vi "Panel.vi"(1 "枚举":enum16{"loop", "back", "advance", "clear"}(ring), 2 "vi reference In":refnum<vi>) -> (0 "vi reference Out":refnum<vi>)   [LabVIEW 2015]
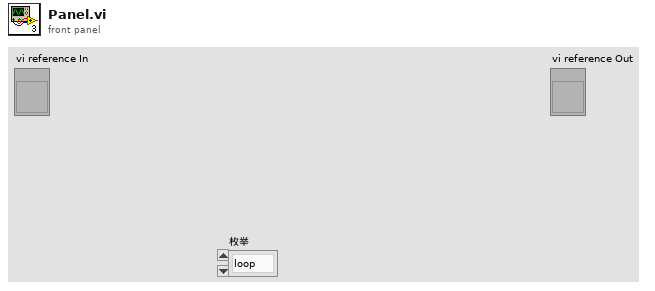
[diagram p1: front panel]
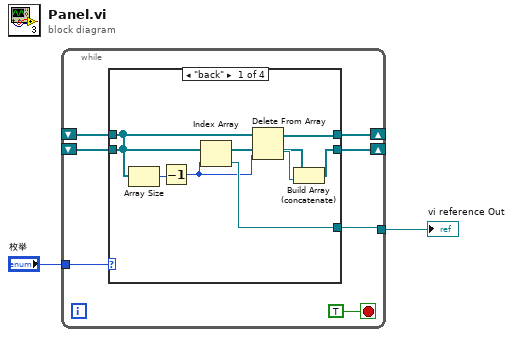
[diagram p0: block diagram]
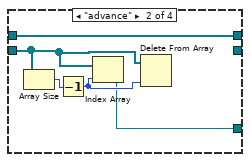
[diagram p2: hidden frame]
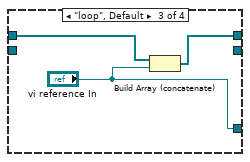
[diagram p3: hidden frame]
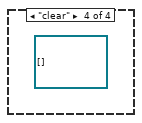
[diagram p4: hidden frame]
diagram:
  n1 = while {
    tunnel: "枚举" -> [w9]
    shift-right: [w7] -> _
    shift-left: _ -> [w6]
    tunnel: [w5] -> w1
    shift-right: [w4] -> _
    shift-left: _ -> [w3]
    stop <- TRUE stop-if-true
    n2 = case shown="\"back\"" w9 {
      tunnel: [w16 w22 w25 _] -> w7
      tunnel: w6 -> [w17 w22 w24 _]
      tunnel: [w15 w18 "vi reference In" _] -> w5
      tunnel: [w12 _ _ _] -> w4
      tunnel: w3 -> [w10 w20 _ _]
      frame "back" {
        n3 = Array Size(array=w17) -> (size(s)=w14:i32)
        n4 = Decrement(x=w14) -> (x-1=w13:i32)
        n5 = Index Array(array=w17, index=w13) -> (element=w15:refnum<vi>)
        n6 = Delete From Array(array=w17, index=w13) -> (deleted portion=w11:refnum<vi>, array with subset deleted=w16:refnum<vi>[])  [unwired: 1 in]
        n7 = Build Array (concatenate)(w10, w11) -> (w12:refnum<vi>[])
      }
      frame "advance" {
        n8 = Array Size(array=w20) -> (size(s)=w21:i32)
        n9 = Decrement(x=w21) -> (x-1=w19:i32)
        n10 = Index Array(array=w20, index=w19) -> (element=w18:refnum<vi>)
        n11 = Delete From Array(array=w20, index=w19) -> ()  [unwired: 1 in, 2 out]
      }
      frame "loop", Default {
        n12 = Build Array (concatenate)(w24, "vi reference In") -> (w25:refnum<vi>[])
      }
      frame "clear" {
        (unwired) refnum<vi>[] []
      }
    }
  }
  "vi reference Out" <- w1
